vi "Inspect Tell Parent.vi"(4 "Priority":bool, 6 "Reply":bool, 8 "Error in":errorcluster, 9 "Msg in":refnum<class "Msg.lvclass">, 11 "Actor in":refnum<class "Actor.lvclass">) -> (0 "Error out":errorcluster, 1 "Msg out":refnum<class "Msg.lvclass">, 2 "Proceed":bool=TRUE, 3 "Actor out":refnum<class "Actor.lvclass">)   [LabVIEW 2020, in "jettl.lvlib" / "Actor.lvclass"]
uses:
  Actor.lvclass
  Msg/Msg.lvclass
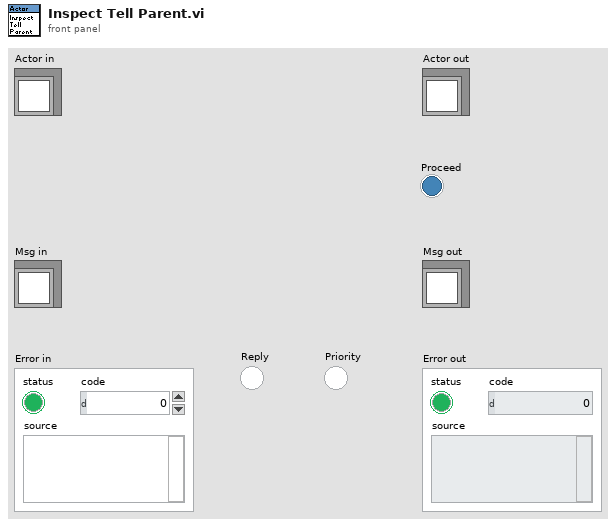
[diagram p1: front panel]
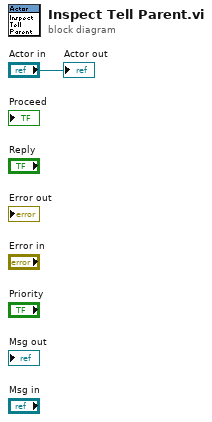
[diagram p0: block diagram]
diagram:
  "Actor out" <- "Actor in"
